vi "Trajectory_Controller.vi"(0 "Error In":errorcluster, 1 "reset":dbl, 5 "Configuration":T1={"Accelerometer Bias"={"X (m/s)"=0.0, "Y (m/s)"=0.0, "Z (m/s)"=0.0}, "Gyroscope Bias"={"X (m/s)"=0.0, "Y (m/s)"=0.0, "Z (m/s)"=0.0}, "Steering Motor Gear Ratio"=611.0, "Steering Pully Gear Ratio"=1.0, "Steering Encoder CPR"=500.0, "Steering Motor Max RPM"=4000.0, "Wheelbase (m)"=1.12, "Fork Angle (rad)"=1.3, "Balancing Controller"={"Kp (/s)"=1.0, "Kd (1)"=1.0}, "Max Allowed Steering Angle (rad)"=0.7, "Task Periods"={"Emergency Stop (us)"=10000, "IMU (us)"=10000, "Steering Motor Encoder (us)"=10000, "State Estimator (us)"=10000, "Balancing Controller (us)"=10000, "GNSS (us)"=10000, "Logging (us)"=50000, "Drive Motor (us)"=100000}, "Drive Motor Gear Ratio"=0.7, "lr"=0.0, "lf"=0.0, "lambda"=0.0, "k1"=0.0, "k2"=0.0, "e1_max"=0.0, "Ad_t"=0.0, "Bd_t"=0.0, "C_t"=0.0, "D_t"=0.0, "Wheel radius"=0.311}, 7 "State Estimate In":refnum<data-value>, 9 "Reset and Init trajectory":bool, 11 "RefTraj in":refnum<data-value>, 12 "Trajectory In":refnum<data-value>, 13 "Measurement In":refnum<data-value>) -> (2 "Measurement Out":refnum<data-value>, 6 "Error out":errorcluster, 10 "Trajectory Out":refnum<data-value>, 14 "Boolean":bool, 15 "Boolean 2":bool)   [LabVIEW 2021]
uses:
  State Estimator/State Estimate.ctl
  Trajectory_Control.ctl
  Configuration/Configuration.ctl
  State Estimator/Measurements.ctl
  IMU/IMU Data.ctl
  Steering Motor Encoder/Steering Motor Encoder Data.ctl
  GNSS/GNSS Data.ctl
panel:
  out "State Estimate In 2":refnum<data-value>
  out "RefTraj out":refnum<data-value>
  out "size(s)":i32[](array[numeric])
  out "error2":dbl
  out "error1":dbl
  out "Rollref":dbl
  out "Closestpoint":dbl
  in  "path in":path=path "libtrajectory_controller.so"
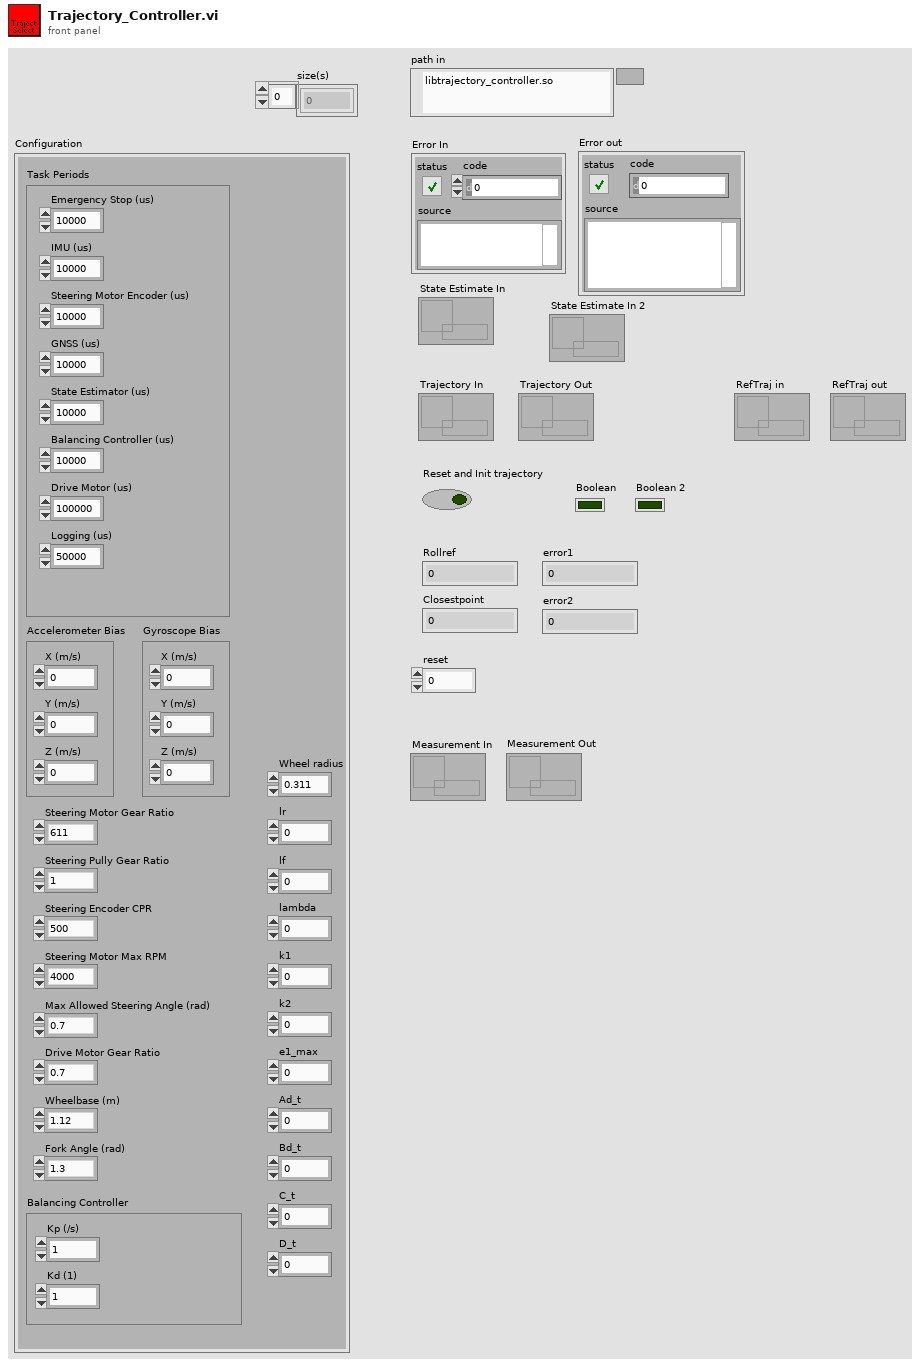
[diagram p1: front panel]
types:
  T1 = typedef "Configuration.ctl" = cluster{"Accelerometer Bias":cluster{"X (m/s)":dbl, "Y (m/s)":dbl, "Z (m/s)":dbl}, "Gyroscope Bias":cluster{"X (m/s)":dbl, "Y (m/s)":dbl, "Z (m/s)":dbl}, "Steering Motor Gear Ratio":dbl, "Steering Pully Gear Ratio":dbl, "Steering Encoder CPR":dbl, "Steering Motor Max RPM":dbl, "Wheelbase (m)":dbl, "Fork Angle (rad)":dbl, "Balancing Controller":cluster{"Kp (/s)":dbl, "Kd (1)":dbl}, "Max Allowed Steering Angle (rad)":dbl, "Task Periods":cluster{"Emergency Stop (us)":i64, "IMU (us)":i64, "Steering Motor Encoder (us)":i64, "State Estimator (us)":i64, "Balancing Controller (us)":i64, "GNSS (us)":i64, "Logging (us)":i64, "Drive Motor (us)":i64}, "Drive Motor Gear Ratio":dbl, "lr":dbl, "lf":dbl, "lambda":dbl, "k1":dbl, "k2":dbl, "e1_max":dbl, "Ad_t":dbl, "Bd_t":dbl, "C_t":dbl, "D_t":dbl, "Wheel radius":dbl}
  T2 = typedef "Trajectory_Control.ctl" = cluster{"Rollref":dbl, "Closestpoint":dbl, "Error1":dbl, "Error2":dbl, "Dpsiref_cont":dbl, "Lateral_cont":dbl, "Heading_cont":dbl, "Reset_traj":dbl, "Iteration":dbl}
  T3 = typedef "Measurements.ctl" = cluster{"IMU Data":T4, "Steering Motor Encoder Data":T5, "GNSS Data":T6}
  T4 = typedef "IMU Data.ctl" = cluster{"Gyroscope":cluster{"X (rad/s)":dbl, "Y (rad/s)":dbl, "Z (rad/s)":dbl}, "Accelerometer":cluster{"X (m/s^2)":dbl, "Y (m/s^2)":dbl, "Z (m/s^2)":dbl}, "Flag IMU":dbl}
  T5 = typedef "Steering Motor Encoder Data.ctl" = cluster{"Encoder Position (counts)":i32, "Steering Angle (rad)":dbl, "Flag Steering Encoder":dbl}
  T6 = typedef "GNSS Data.ctl" = cluster{"Latitude (rad)":dbl, "Longitude (rad)":dbl, "Altitude (m)":dbl, "Speed (m/s)":dbl, "Heading (rad)":dbl, "Fix Quality":i32, "Number of Satellites":i32, "Latitude (deg)":dbl, "Longitude (deg)":dbl, "Flag GNSS":dbl}
  T7 = typedef "State Estimate.ctl" = cluster{"X (m)":dbl, "Y (m)":dbl, "Psi (rad)":dbl, "Roll (rad)":dbl, "Roll Rate (rad/s)":dbl, "delta":dbl, "velocity":dbl, "Iterations":dbl}
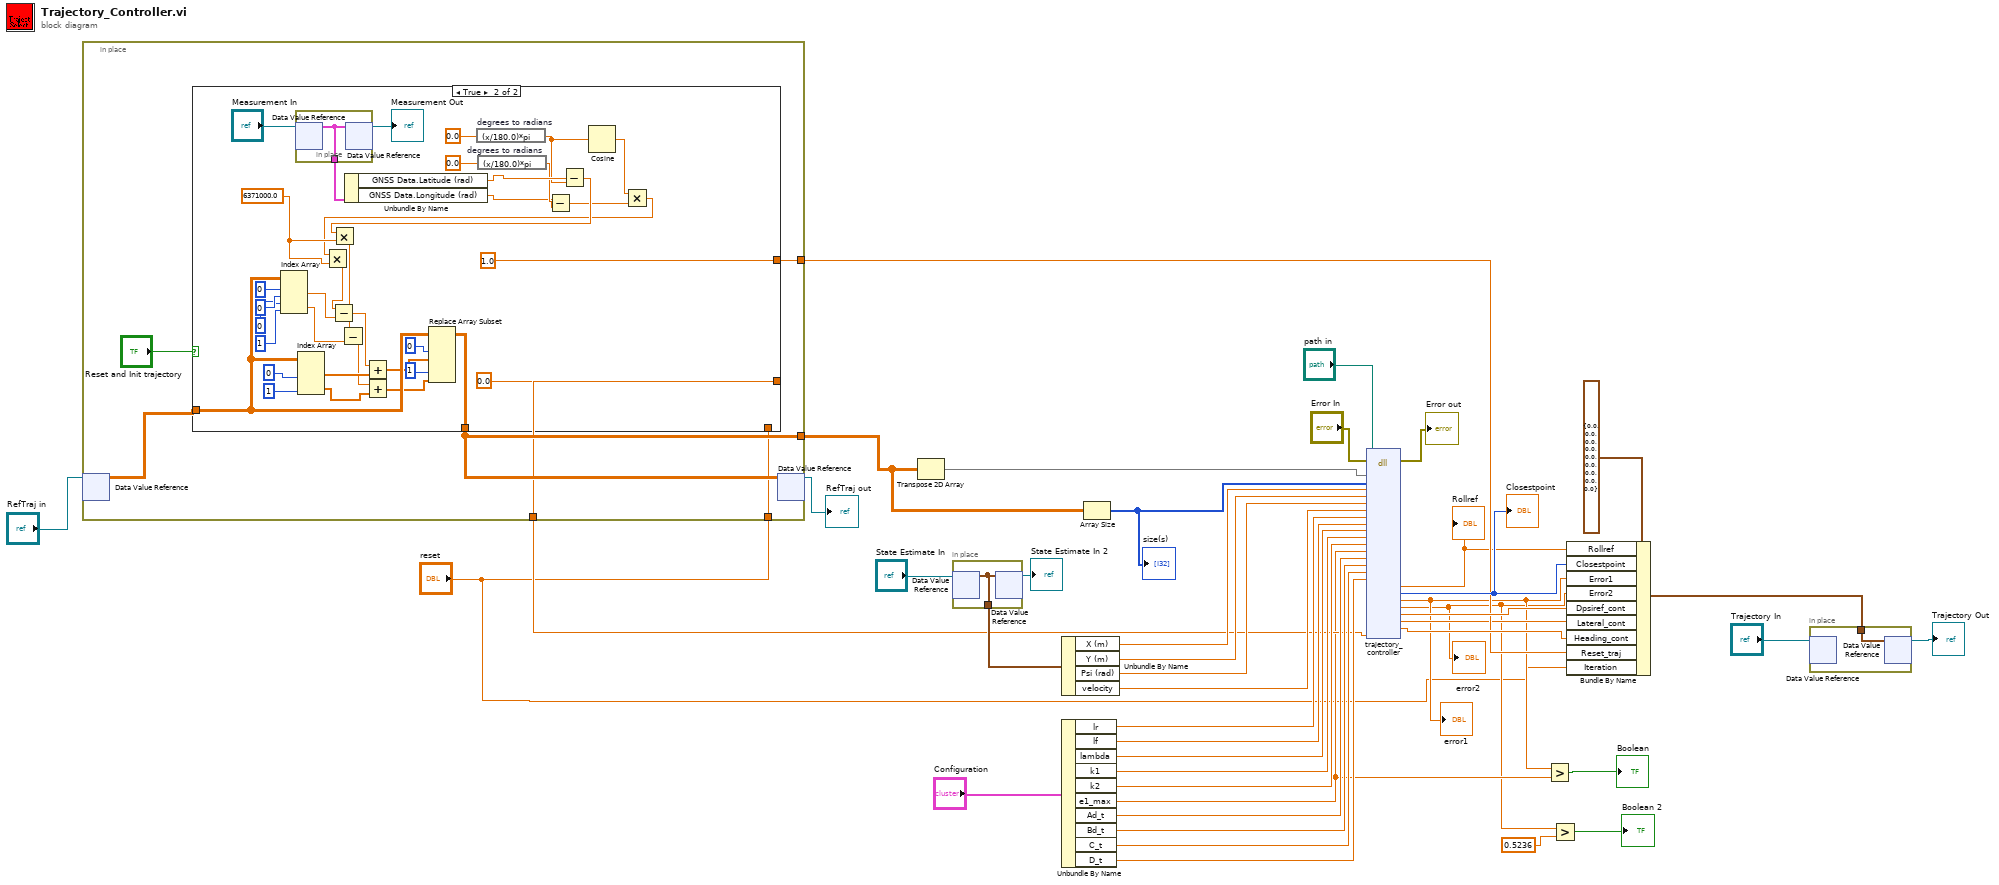
[diagram p0: block diagram]
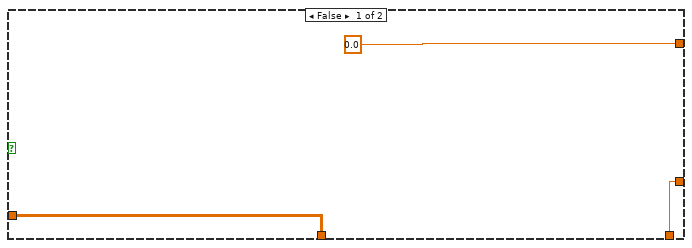
[diagram p2: hidden frame]
diagram:
  n1 = in-place {
    in-place-border: [w47] -> w10
    in-place-border: [w49] -> w13
    in-place-border: [w45] -> w12
    in-place-border: "reset" -> [w44]
    n2 = in-place-dvr #1("RefTraj in") -> (w48:dbl[][])  [unwired: 1 out]
    n3 = case shown="True" "Reset and Init trajectory" {
      tunnel: [w50 0.0] -> w47
      tunnel: [w52 w70] -> w49
      tunnel: w48 -> [w52 w80]
      tunnel: [0.0 1.0] -> w45
      tunnel: w44 -> [w50 _]
      frame False {
      }
      frame True {
        w82 = 6371000.0
        n4 = Index Array(array=w80, index (row) #1=0, index (col) #1=0, index (row) #2=0, index (col) #2=1) -> (element #1=w53:dbl, element #2=w75:dbl)
        n5 = in-place {
          in-place-border: [w89] -> w85
          n6 = in-place-dvr #2("Measurement In") -> (w89:T3)  [unwired: 1 out]
          n7 = in-place-dvr #2(w89) -> (→"Measurement Out":refnum<data-value>)  [unwired: 1 out]
        }
        n8 = Index Array(array=w80, index (col) #1=0, index (col) #2=1) -> (element #1=w83:dbl[], element #2=w72:dbl[])  [unwired: 2 in]
        n9 = Unbundle By Name(w85) -> ("GNSS Data.Latitude (rad)"=w64:dbl, "GNSS Data.Longitude (rad)"=w60:dbl)
        n10 = expression code="(x/180.0)*pi" "degrees to radians"(0.0 ("y")) -> (w58:dbl)
        n11 = expression code="(x/180.0)*pi" "degrees to radians"(0.0 ("y")) -> (w61:dbl)
        n12 = Subtract(x=w60, y=w61) -> (x-y=w56:dbl)
        n13 = Subtract(x=w64, y=w58) -> (x-y=w59:dbl)
        n14 = Multiply(x=w59, y=w82) -> (x*y=w81:dbl)
        n15 = Subtract(x=w81, y=w75) -> (x-y=w73:dbl)
        n16 = Add(x=w73, y=w72) -> (x+y=w71:dbl[])
        n17 = Cosine(x=w58) -> (cos(x)=w57:dbl)
        n18 = Multiply(x=w57, y=w56) -> (x*y=w55:dbl)
        n19 = Multiply(x=w55, y=w82) -> (x*y=w54:dbl)
        n20 = Subtract(x=w54, y=w53) -> (x-y=w84:dbl)
        n21 = Add(x=w84, y=w83) -> (x+y=w74:dbl[])
        n22 = Replace Array Subset(array=w80, new element #1=w74, index (col) #1=0, new element #2=w71, index (col) #2=1) -> (w70:dbl[][])  [unwired: 2 in]
      }
    }
    n23 = in-place-dvr #1(w49) -> (→"RefTraj out":refnum<data-value>)  [unwired: 1 out]
  }
  n24 = Transpose 2D Array(2D array=w13) -> (transposed array=w14:dbl[][])
  n25 = in-place {
    in-place-border: [w90] -> w41
    n26 = in-place-dvr #3("State Estimate In") -> (w90:T7)  [unwired: 1 out]
    n27 = in-place-dvr #3(w90) -> (→"State Estimate In 2":refnum<data-value>)  [unwired: 1 out]
  }
  n28 = Unbundle By Name(w41) -> ("X (m)"=w40:dbl, "Y (m)"=w39:dbl, "Psi (rad)"=w38:dbl, "velocity"=w22:dbl)
  n29 = Unbundle By Name("Configuration") -> ("lr"=w31:dbl, "lf"=w30:dbl, "lambda"=w29:dbl, "k1"=w28:dbl, "k2"=w27:dbl, "e1_max"=w6:dbl, "Ad_t"=w26:dbl, "Bd_t"=w25:dbl, "C_t"=w24:dbl, "D_t"=w23:dbl)
  n30 = Array Size(array=w13) -> (size(s)=w15:i32[])
  "size(s)" <- w15
  n31 = dll-call lib="libtrajectory_controller.so" fn="trajectory_controller"(path in="path in", error in="Error In", "Traj"=w14, "traj_size"=w15, "X"=w40, "Y"=w39, "Psi"=w38, "v"=w22, "lr"=w31, "lf"=w30, "lambda"=w29, "k1"=w28, "k2"=w27, "e1max"=w6, "Adt"=w26, "Bdt"=w25, "Ct"=w24, "Dt"=w23, "Reset"=w10) -> (error out=→"Error out":errorcluster, "Rollref"=w9:dbl, "Closestpoint"=w20:i32, "error1"=w5:dbl, "error2"=w3:dbl, "dpsiref_cont"=w19:dbl, "Lateral_cont"=w8:dbl, "Heading_cont"=w18:dbl)  [unwired: 26 in, 1 out]
  "Closestpoint" <- w20
  "Rollref" <- w9
  "error1" <- w5
  "error2" <- w3
  n32 = Greater?(x=w5, y=w6) -> (0:→"Boolean":bool)
  n33 = Greater?(x=w3, y=0.5236) -> (0:→"Boolean 2":bool)
  n34 = Bundle By Name(cluster=T2 {"Rollref"=0.0, "Closestpoint"=0.0, "Error1"=0.0, "Error2"=0.0, "Dpsiref_cont"=0.0, "Lateral_cont"=0.0, "Heading_cont"=0.0, "Reset_traj"=0.0, "Iteration"=0.0} ("Trajectory (Debug)"), "Rollref"=w9, "Closestpoint"=w20, "Error1"=w5, "Error2"=w3, "Dpsiref_cont"=w19, "Lateral_cont"=w8, "Heading_cont"=w18, "Reset_traj"=w12, "Iteration"="reset") -> (w33:T2)
  n35 = in-place {
    in-place-border: w33 -> [w91]
    n36 = in-place-dvr #4("Trajectory In") -> ()  [unwired: 2 out]
    n37 = in-place-dvr #4(w91) -> (→"Trajectory Out":refnum<data-value>)  [unwired: 1 out]
  }
